vi "Arduino+excel.vi"() -> ()   [LabVIEW 2019]
uses:
  <vilib>/Utility/file.llb/Write Delimited Spreadsheet (string).vi
panel:
  in  "file path (dialog if empty)":path
  out "Array":string[](array[string])
  in  "stop":bool
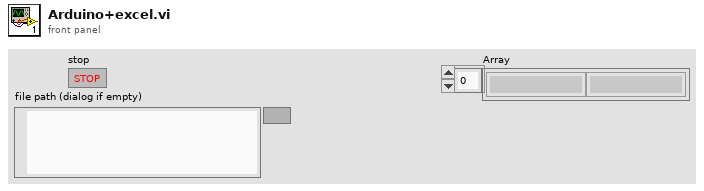
[diagram p1: front panel]
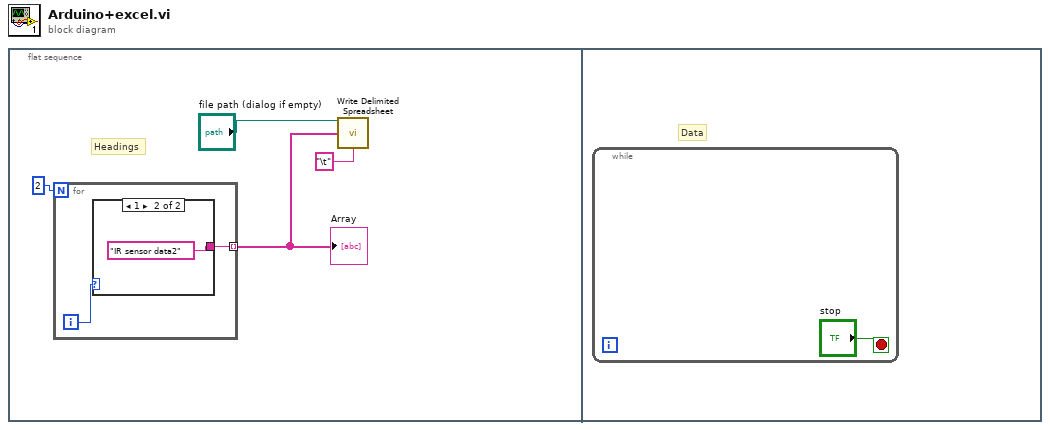
[diagram p0: block diagram]
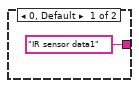
[diagram p2: hidden frame]
diagram:
  n1 = flat-sequence {
    frame #0 {
      # "Headings"
      n2 = for {
        N: 2 -> [_]
        tunnel: [w5] -> w2 mode=indexing
        i -> [w6]
        n3 = case shown="1" w6 {
          tunnel: ["IR sensor data1" "IR sensor data2"] -> w5
          frame 0, Default {
          }
          frame 1 {
          }
        }
      }
      "Array" <- w2
      n4 = call-poly <vilib>:"Write Delimited Spreadsheet.vi"("file path (dialog if empty)"="file path (dialog if empty)", "1D data"=w2, "delimiter (\\t)"="\t" ("delimiter (\\t)")) -> ()  [unwired: 11 in, 2 out]
    }
    frame #1 {
      # "Data"
      n5 = while {
        stop <- "stop" stop-if-true
      }
    }
  }
